vi "[Debug] Observe Multiplier FIFO.vi"(0 "Boolean":bool) -> (1 "Mult":fxp<+/-,18,1>[](array[numeric]) format="%.18g", 2 "Args":u8[](array[numeric]), 3 "Ident":u8[](array[numeric]))   [LabVIEW 2009]
uses:
  <vilib>/rvi/DataTransferAndStorage/Container/XNode/niFpgaContainer.xnode
  <vilib>/rvi/DataTransferAndStorage/Container/Common/niFpgaContainerExecOnDevCompGetState.vi
  <vilib>/rvi/DataTransferAndStorage/Container/Common/niFpgaContainerMetaDataKey.ctl
  <vilib>/rvi/Memory/Memory_Emulation/nirvimemoryEmulationManagerCache_GetValue.vi
  <vilib>/rvi/Memory/Memory_Emulation/nirvimemoryEmulationManagerCache_InsertValue.vi
  <vilib>/rvi/FIFO/Fifo_Resource/nirvififoUniquifyingName.vi
  <vilib>/Utility/error.llb/Clear Errors.vi
  <vilib>/rvi/Memory/Memory_Emulation/nirvimemoryEmulationManagerCache_SetValue.vi
panel:
  out "Done Update":bool=TRUE
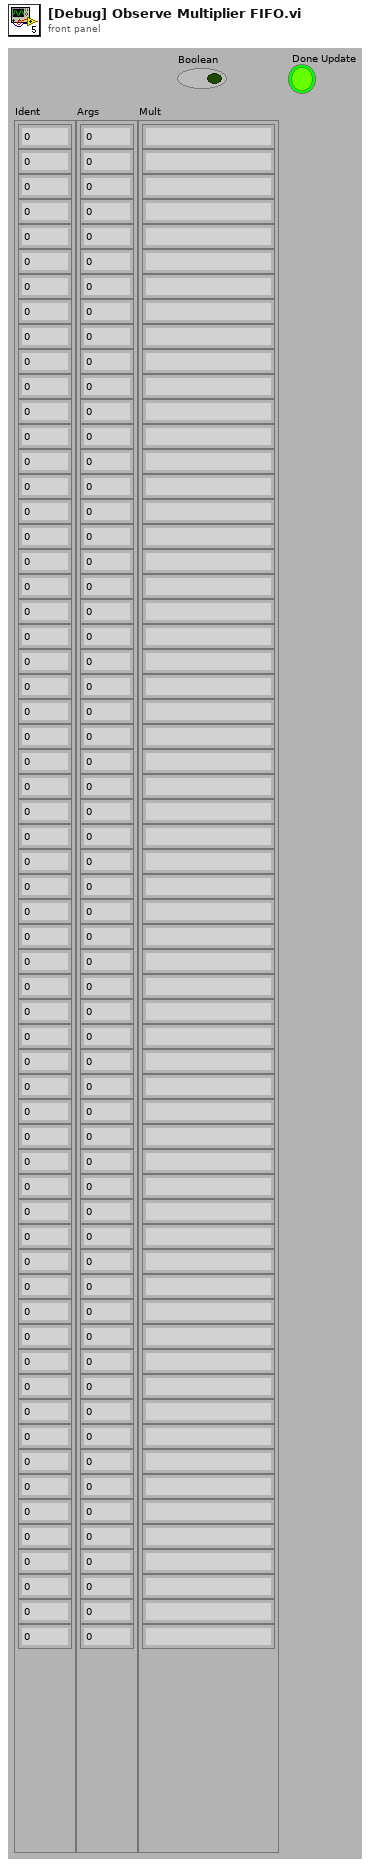
[diagram p1: front panel]
types:
  T1 = typedef "niFpgaContainerMetaDataKey.ctl" = enum16{"FPGA FIFO", "FPGA Memory", "FPGA Register"}
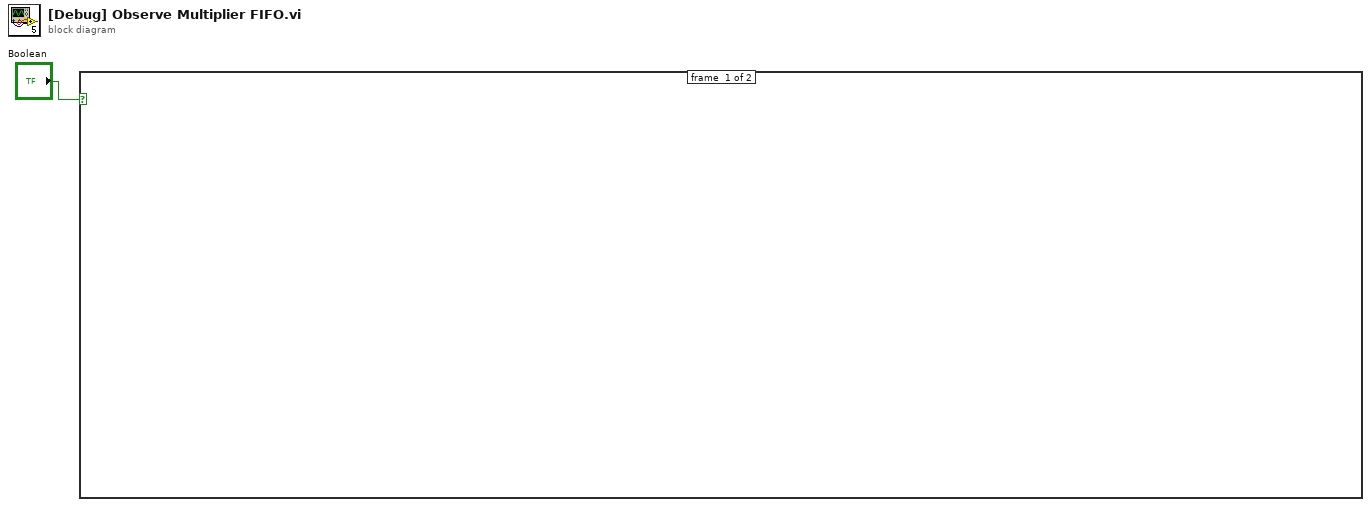
[diagram p0: block diagram]
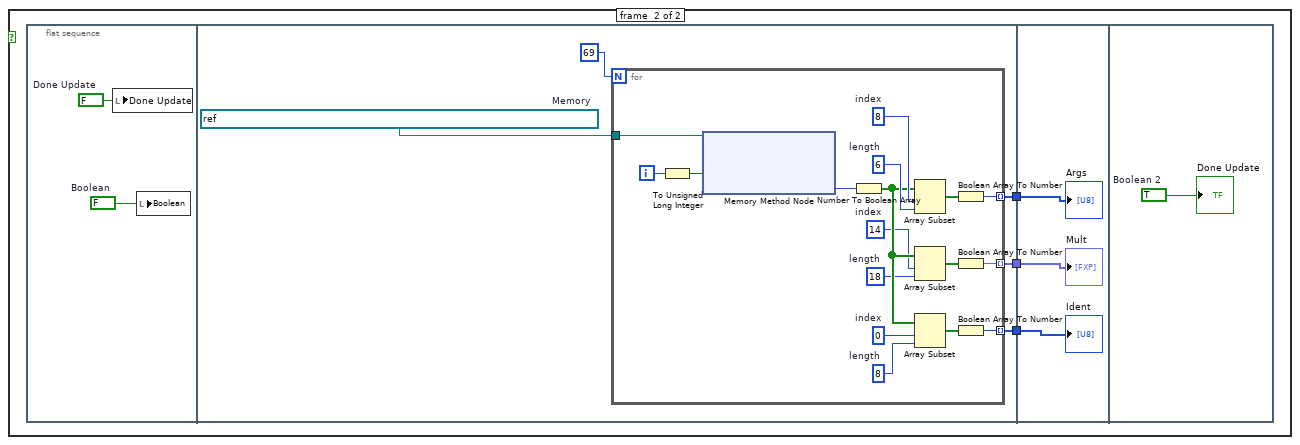
[diagram p2: hidden frame]
diagram:
  n1 = case shown="True" "Boolean" {
    frame #0 {
    }
    frame #1 {
      n2 = flat-sequence {
        tunnel: [w11] -> w4
        tunnel: [w10] -> w3
        tunnel: [w9] -> w2
        tunnel: w4 -> [w197]
        tunnel: w3 -> [w198]
        tunnel: w2 -> [w196]
        frame #0 {
          w5 = FALSE  # Done Update
          w6 = FALSE  # Boolean
          n3 = local write "Done Update"(w5) -> ()
          n4 = local write "Boolean"(w6) -> ()
        }
        frame #1 {
          w8 = refnum<k21> "Multiplier 1 Block Memory Out : [8b Identifier; 6b args; 18b fxp output]"  # Memory
          n5 = for {
            N: 69 -> [_]
            tunnel: w8 -> [w28]
            tunnel: [w15] -> w9 mode=indexing
            tunnel: [w13] -> w11 mode=indexing
            tunnel: [w12] -> w10 mode=indexing
            i -> [w27]
            w19 = 18  # length
            w20 = 14  # index
            w22 = 6  # length
            w23 = 8  # index
            w24 = 8  # length
            w25 = 0  # index
            n6 = To Unsigned Long Integer(number=w27) -> (unsigned 32bit integer=w26:u32)
            n7 = xnode ("Memory Method Node")("Address"=w26, "Memory In"=w28) -> ("Data"=w17:u32)  [unwired: 1 out]
            n8 = Number To Boolean Array(number=w17) -> (Boolean array=w21:bool[])
            n9 = Array Subset(array=w21, index=w23, length=w22) -> (w14:bool[])
            n10 = Array Subset(array=w21, index=w20, length=w19) -> (w18:bool[])
            n11 = Array Subset(array=w21, index=w25, length=w24) -> (w16:bool[])
            n12 = Boolean Array To Number(Boolean array=w14) -> (number=w12:u8)
            n13 = Boolean Array To Number(Boolean array=w18) -> (number=w13:fxp<+/-,18,1>)
            n14 = Boolean Array To Number(Boolean array=w16) -> (number=w15:u8)
          }
        }
        frame #2 {
          "Mult" <- w197
          "Args" <- w198
          "Ident" <- w196
        }
        frame #3 {
          w199 = TRUE  # Boolean 2
          "Done Update" <- w199
        }
      }
    }
  }
